vi "Is Error.vi"(11 "Base Queue jettl in":refnum<class "Base Queue jettl.lvclass">) -> (3 "Base Queue jettl out":refnum<class "Base Queue jettl.lvclass">)   [LabVIEW 2021, in "jettl.lvlib" / "Base Queue jettl.lvlib" / "Base Queue jettl.lvclass"]
uses:
  Base Queue jettl.lvclass
  State/Error State/Error State.lvclass
  C:/git/jettl/src/jettl/Base Queue jettl/State/State/State.lvclass
  Base Queue jettl.lvclass/Base Queue jettl.ctl
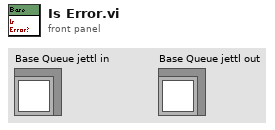
[diagram p1: front panel]
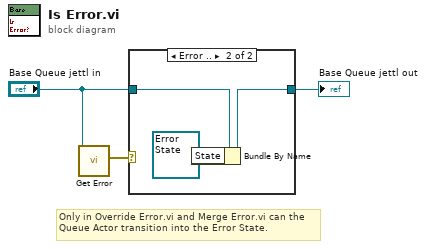
[diagram p0: block diagram]
diagram:
  # "Only in Override Error.vi and Merge Error.vi can the Queue Actor transition into the Error State."
  n1 = call-dynamic "Get Error.vi"("Base Queue jettl in"="Base Queue jettl in") -> ("Error"=w3:errorcluster)  [unwired: 10 in]
  n2 = case shown="Error .." w3 {
    tunnel: [w4 w6] -> w1
    tunnel: "Base Queue jettl in" -> [w4 w7]
    frame No Error {
    }
    frame Error {
      n3 = Bundle By Name(cluster=w7, "State"=refnum<class "Error State.lvclass"> refnum ("jettl.lvlib:jettl Queue Actor.lvlib:Error State.lvclass")) -> (w6:refnum<class "Base Queue jettl.lvclass">)
    }
  }
  "Base Queue jettl out" <- w1
